vi "Make Impulse Array.vi"(8 "error in (no error)":errorcluster, 11 "Class out":refnum<class "Impulse Data.lvclass">) -> (0 "error out":errorcluster, 3 "Class In":refnum<class "Impulse Data.lvclass">)   [LabVIEW 2016, in "Impulse Data.lvclass"]
uses:
  Impulse Data.lvclass
  Impulse Data.lvclass/Impulse Data.ctl
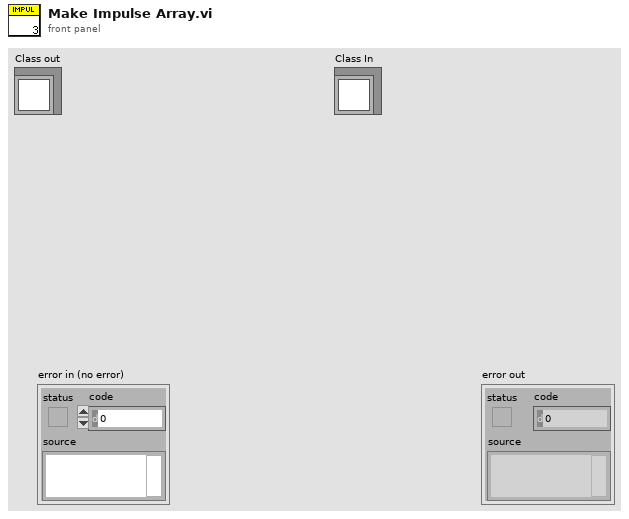
[diagram p1: front panel]
types:
  T1 = typedef "TD_Impulse Planes.ctl" = enum16{"Other", "Yaw", "Pitch", "Roll", "LARP", "RALP"}
  T2 = cluster{"Impulse Plane":T1, "Impulse Direction +ve?":bool, "Start":i32, "Duration":i32}[]
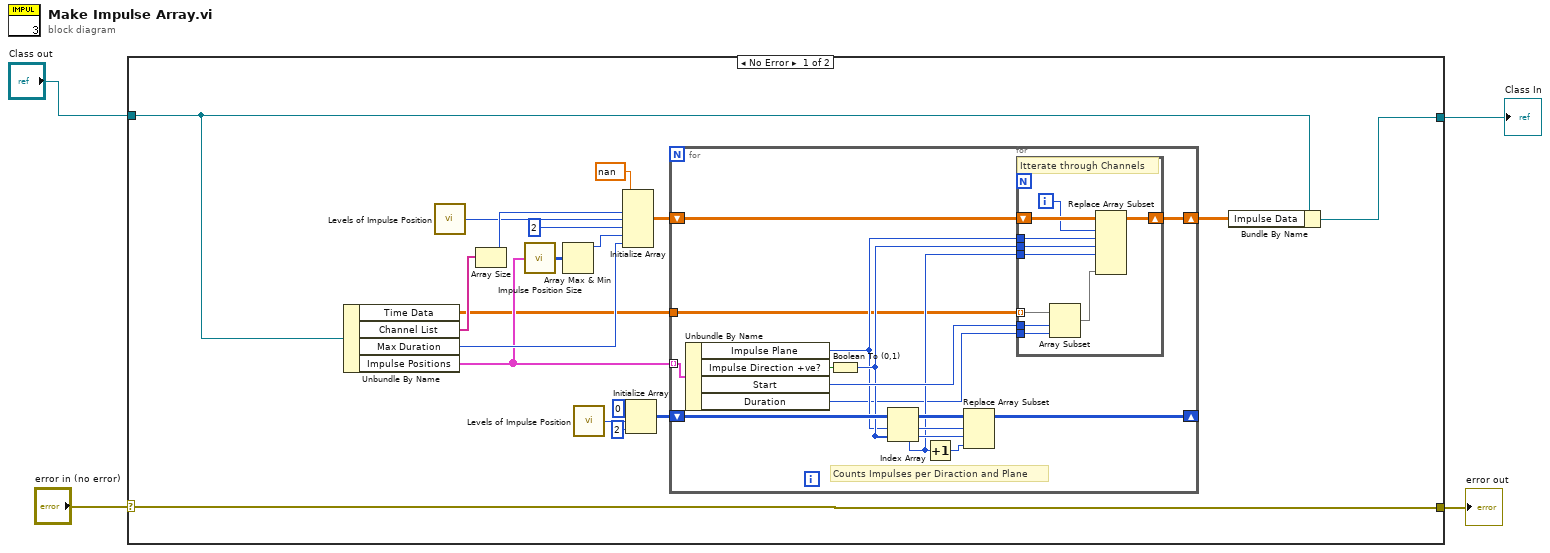
[diagram p0: block diagram]
diagram:
  n1 = case shown="No Error" "error in (no error)" {
    selector: "error in (no error)" -> [w23 w48]
    tunnel: [w23 w48] -> w3
    tunnel: "Class out" -> [w6 w47]
    tunnel: [w5 w47] -> w1
    frame No Error {
      n2 = Unbundle By Name(w6) -> ("Time Data"=w8:dbl[][], "Channel List"=w20:string[], "Max Duration"=w22:i32, "Impulse Positions"=w21:T2)
      n3 = call "Levels of Impulse Position.vi"() -> ("Size"=w16:i32)  [unwired: 1 in]
      n4 = Array Size(array=w20) -> (size(s)=w18:i32)
      n5 = call "Impulse Position Size.vi"("Impulse Positions"=w21) -> ("Impulse Position size"=w15:i32[][])
      n6 = Array Max & Min(array=w15) -> (max value=w14:i32)  [unwired: 3 out]
      n7 = call "Levels of Impulse Position.vi"() -> ("Size"=w11:i32)  [unwired: 1 in]
      n8 = Initialize Array(nan ("element"), w18, w16, 2 ("dimension size"), w14, w22) -> (w13:dbl[][][][][])
      n9 = Initialize Array(0, w11, 2 ("dimension size")) -> (w12:i32[][])
      n10 = for {
        tunnel: w21 -> [w33] mode=indexing
        shift-right: [w35] -> w7
        shift-left: w13 -> [w36]
        shift-right: [w25] -> _
        shift-left: w12 -> [w30]
        tunnel: w8 -> [w24]
        # "Counts Impulses per Diraction and Plane"
        n11 = Unbundle By Name(w33) -> ("Impulse Plane"=w28:T1, "Impulse Direction +ve?"=w32:bool, "Start"=w34:i32, "Duration"=w26:i32)
        n12 = Boolean To (0,1)(Boolean=w32) -> (0, 1=w29:i16)
        n13 = Index Array(array=w30, index (row)=w28, index (col)=w29) -> (element=w27:i32)
        n14 = Increment(x=w27) -> (x+1=w31:i32)
        n15 = Replace Array Subset(array=w30, new element=w31, index (row)=w28, index (col)=w29) -> (w25:i32[][])
        n16 = for {
          tunnel: w24 -> [w38] mode=indexing
          tunnel: w34 -> [w44]
          tunnel: w29 -> [w43]
          tunnel: w28 -> [w42]
          tunnel: w27 -> [w41]
          tunnel: w26 -> [w40]
          shift-right: [w45] -> w35
          shift-left: w36 -> [w46]
          i -> [w39]
          # "Itterate through Channels"
          n17 = Array Subset(array=w38, index=w44, length=w40) -> (w37:dbl[])
          n18 = Replace Array Subset(array=w46, new element=w37, index (dim 0)=w39, index (dim 1)=w42, index (dim 2)=w43, index (dim 3)=w41) -> (w45:dbl[][][][][])  [unwired: 1 in]
        }
      }
      n19 = Bundle By Name(cluster=w6, "Impulse Data"=w7) -> (w5:refnum<class "Impulse Data.lvclass">)
    }
    frame Error {
    }
  }
  "error out" <- w3
  "Class In" <- w1
